vi "value to Rcode.vi"(9 "Manual Range (0)":dbl format="%#_6p", 11 "Function (1: DC Volts)":u16(ring)=1 items=["DC Volts"=1, "AC Volts"=2, "2-Wire Resistance"=3, "4-Wire Resistance"=4, "DC Current"=5, "AC Current"=6, "(AC + DC) Volts"=7, "(AC + DC) Current"=8, "DCV Bch"=12, "Diode"=13, "2-Wire Resistance( Low-Power)"=20, "4-Wire Resistance( Low-Power)"=21, "Continuity"=22, "Frequency"=50]) -> (2 "Range Set Code":string)   [LabVIEW 2020, in "ADCMT7451_ADC.lvlib"]
uses:
  ADCMT7451_ADC.lvlib
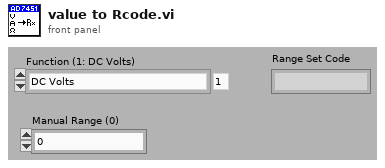
[diagram p1: front panel]
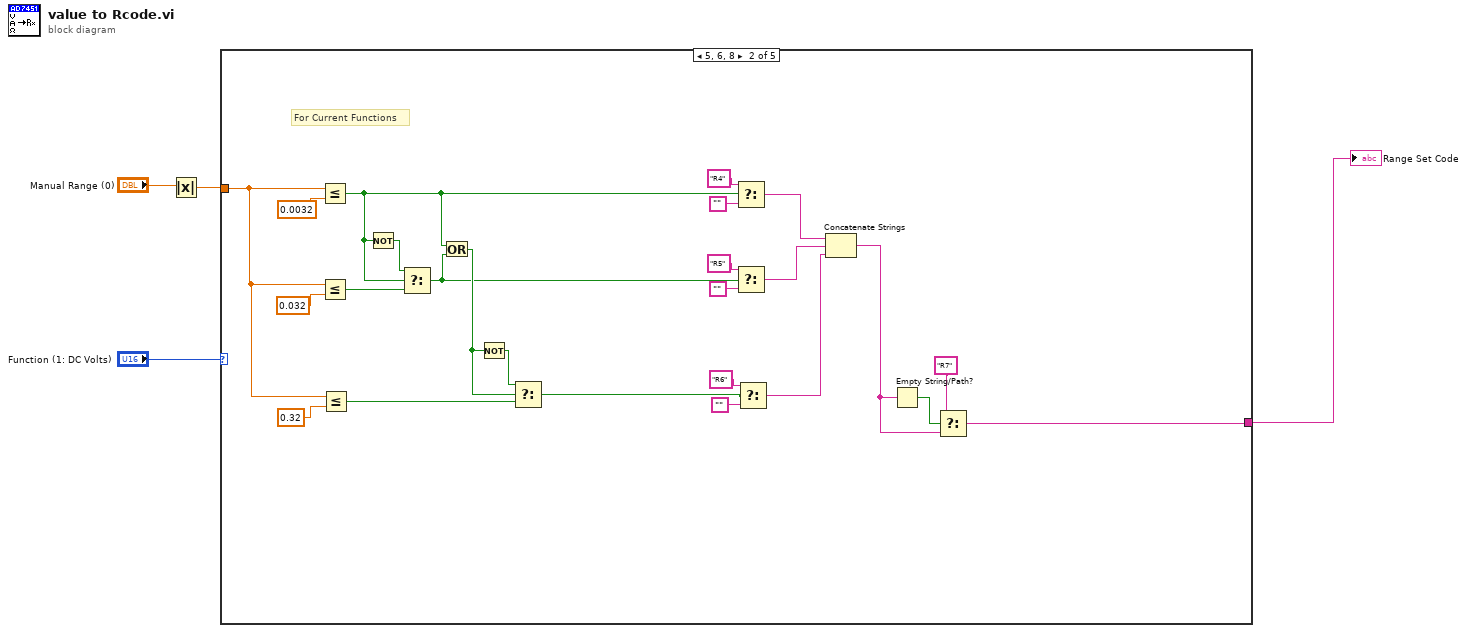
[diagram p0: block diagram]
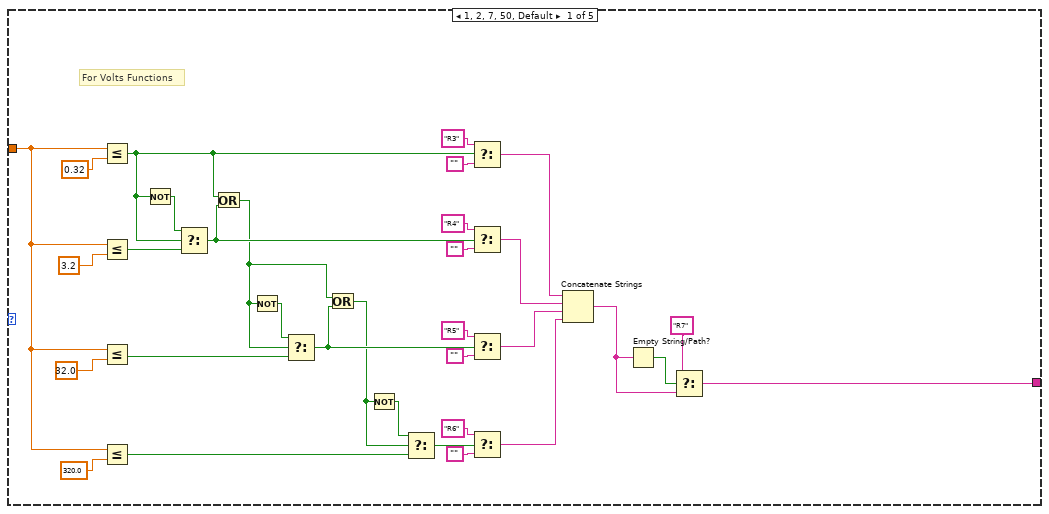
[diagram p2: hidden frame]
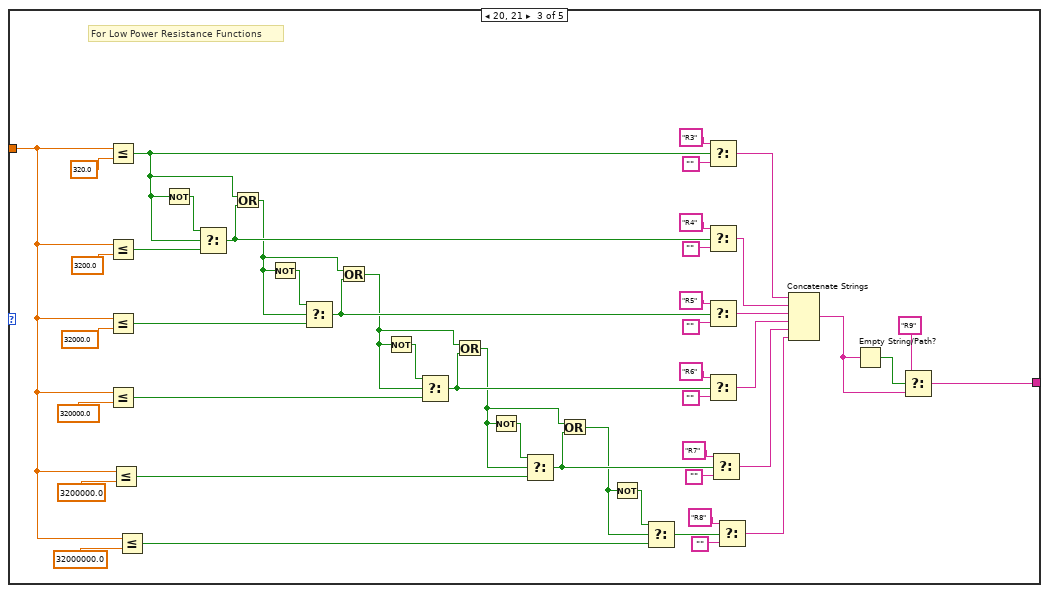
[diagram p3: hidden frame]
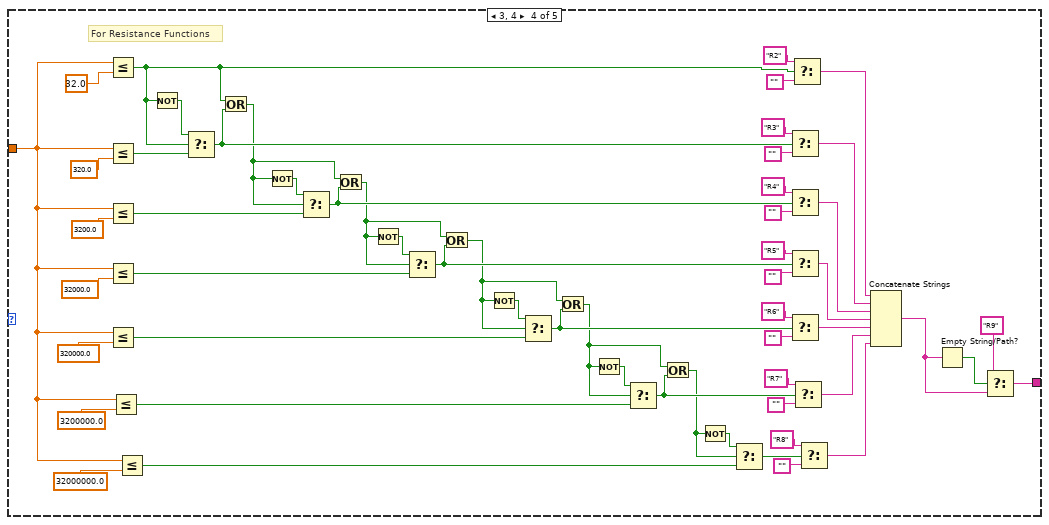
[diagram p4: hidden frame]
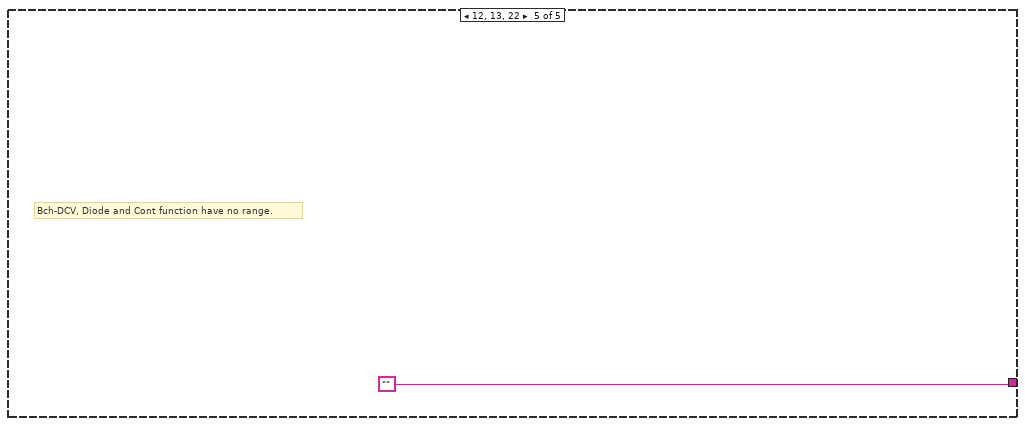
[diagram p5: hidden frame]
diagram:
  n1 = Absolute Value(x="Manual Range (0)") -> (abs(x)=w2:dbl)
  n2 = case shown="5, 6, 8" "Function (1: DC Volts)" {
    tunnel: w2 -> [w25 w42 w64 w121 _]
    tunnel: [w17 w51 w93 w151 ""] -> w3
    frame 1, 2, 7, 50, Default {
      # "For Volts Functions"
      n3 = Less Or Equal?(x=w25, y=0.32) -> (x <= y?=w9:bool)
      n4 = Less Or Equal?(x=w25, y=3.2) -> (x <= y?=w16:bool)
      n5 = Less Or Equal?(x=w25, y=32.0) -> (x <= y?=w13:bool)
      n6 = Less Or Equal?(x=w25, y=320.0) -> (x <= y?=w11:bool)
      n7 = Not(x=w9) -> (.not. x?=w15:bool)
      n8 = Select(t=w15, s=w9, f=w16) -> (s? t:f=w8:bool)
      n9 = Or(x=w9, y=w8) -> (x .or. y?=w5:bool)
      n10 = Not(x=w5) -> (.not. x?=w14:bool)
      n11 = Select(t=w14, s=w5, f=w13) -> (s? t:f=w7:bool)
      n12 = Or(x=w5, y=w7) -> (x .or. y?=w6:bool)
      n13 = Not(x=w6) -> (.not. x?=w12:bool)
      n14 = Select(t=w12, s=w6, f=w11) -> (s? t:f=w10:bool)
      n15 = Select(t="R3", s=w9, f="") -> (s? t:f=w24:string)
      n16 = Select(t="R4", s=w8, f="") -> (s? t:f=w23:string)
      n17 = Select(t="R5", s=w7, f="") -> (s? t:f=w22:string)
      n18 = Select(t="R6", s=w10, f="") -> (s? t:f=w21:string)
      n19 = Concatenate Strings(w24, w23, w22, w21) -> (w18:string)
      n20 = Empty String/Path?(string/path=w18) -> (empty?=w20:bool)
      n21 = Select(t="R7", s=w20, f=w18) -> (s? t:f=w17:string)
    }
    frame 5, 6, 8 {
      # "For Current Functions"
      n22 = Less Or Equal?(x=w42, y=0.0032) -> (x <= y?=w46:bool)
      n23 = Less Or Equal?(x=w42, y=0.032) -> (x <= y?=w49:bool)
      n24 = Less Or Equal?(x=w42, y=0.32) -> (x <= y?=w43:bool)
      n25 = Not(x=w46) -> (.not. x?=w50:bool)
      n26 = Select(t=w50, s=w46, f=w49) -> (s? t:f=w45:bool)
      n27 = Or(x=w46, y=w45) -> (x .or. y?=w47:bool)
      n28 = Not(x=w47) -> (.not. x?=w48:bool)
      n29 = Select(t=w48, s=w47, f=w43) -> (s? t:f=w39:bool)
      n30 = Select(t="R4", s=w46, f="") -> (s? t:f=w56:string)
      n31 = Select(t="R5", s=w45, f="") -> (s? t:f=w55:string)
      n32 = Select(t="R6", s=w39, f="") -> (s? t:f=w38:string)
      n33 = Concatenate Strings(w56, w55, w38) -> (w52:string)
      n34 = Empty String/Path?(string/path=w52) -> (empty?=w54:bool)
      n35 = Select(t="R7", s=w54, f=w52) -> (s? t:f=w51:string)
    }
    frame 20, 21 {
      # "For Low Power Resistance Functions"
      n36 = Less Or Equal?(x=w64, y=320.0) -> (x <= y?=w63:bool)
      n37 = Less Or Equal?(x=w64, y=3200.0) -> (x <= y?=w82:bool)
      n38 = Less Or Equal?(x=w64, y=32000.0) -> (x <= y?=w80:bool)
      n39 = Less Or Equal?(x=w64, y=320000.0) -> (x <= y?=w78:bool)
      n40 = Less Or Equal?(x=w64, y=3200000.0) -> (x <= y?=w74:bool)
      n41 = Less Or Equal?(x=w64, y=32000000.0) -> (x <= y?=w71:bool)
      n42 = Not(x=w63) -> (.not. x?=w83:bool)
      n43 = Select(t=w83, s=w63, f=w82) -> (s? t:f=w77:bool)
      n44 = Or(x=w63, y=w77) -> (x .or. y?=w67:bool)
      n45 = Not(x=w67) -> (.not. x?=w81:bool)
      n46 = Select(t=w81, s=w67, f=w80) -> (s? t:f=w76:bool)
      n47 = Or(x=w67, y=w76) -> (x .or. y?=w66:bool)
      n48 = Not(x=w66) -> (.not. x?=w79:bool)
      n49 = Select(t=w79, s=w66, f=w78) -> (s? t:f=w68:bool)
      n50 = Or(x=w66, y=w68) -> (x .or. y?=w65:bool)
      n51 = Not(x=w65) -> (.not. x?=w75:bool)
      n52 = Select(t=w75, s=w65, f=w74) -> (s? t:f=w73:bool)
      n53 = Or(x=w65, y=w73) -> (x .or. y?=w69:bool)
      n54 = Not(x=w69) -> (.not. x?=w72:bool)
      n55 = Select(t=w72, s=w69, f=w71) -> (s? t:f=w70:bool)
      n56 = Select(t="R3", s=w63, f="") -> (s? t:f=w99:string)
      n57 = Select(t="R4", s=w77, f="") -> (s? t:f=w98:string)
      n58 = Select(t="R5", s=w76, f="") -> (s? t:f=w97:string)
      n59 = Select(t="R6", s=w68, f="") -> (s? t:f=w86:string)
      n60 = Select(t="R7", s=w73, f="") -> (s? t:f=w84:string)
      n61 = Select(t="R8", s=w70, f="") -> (s? t:f=w85:string)
      n62 = Concatenate Strings(w99, w98, w97, w86, w84, w85) -> (w94:string)
      n63 = Empty String/Path?(string/path=w94) -> (empty?=w96:bool)
      n64 = Select(t="R9", s=w96, f=w94) -> (s? t:f=w93:string)
    }
    frame 3, 4 {
      # "For Resistance Functions"
      n65 = Less Or Equal?(x=w121, y=32.0) -> (x <= y?=w115:bool)
      n66 = Less Or Equal?(x=w121, y=320.0) -> (x <= y?=w119:bool)
      n67 = Less Or Equal?(x=w121, y=3200.0) -> (x <= y?=w140:bool)
      n68 = Less Or Equal?(x=w121, y=32000.0) -> (x <= y?=w138:bool)
      n69 = Less Or Equal?(x=w121, y=320000.0) -> (x <= y?=w136:bool)
      n70 = Less Or Equal?(x=w121, y=3200000.0) -> (x <= y?=w132:bool)
      n71 = Less Or Equal?(x=w121, y=32000000.0) -> (x <= y?=w129:bool)
      n72 = Not(x=w115) -> (.not. x?=w120:bool)
      n73 = Select(t=w120, s=w115, f=w119) -> (s? t:f=w116:bool)
      n74 = Or(x=w115, y=w116) -> (x .or. y?=w114:bool)
      n75 = Not(x=w114) -> (.not. x?=w141:bool)
      n76 = Select(t=w141, s=w114, f=w140) -> (s? t:f=w135:bool)
      n77 = Or(x=w114, y=w135) -> (x .or. y?=w125:bool)
      n78 = Not(x=w125) -> (.not. x?=w139:bool)
      n79 = Select(t=w139, s=w125, f=w138) -> (s? t:f=w134:bool)
      n80 = Or(x=w125, y=w134) -> (x .or. y?=w124:bool)
      n81 = Not(x=w124) -> (.not. x?=w137:bool)
      n82 = Select(t=w137, s=w124, f=w136) -> (s? t:f=w126:bool)
      n83 = Or(x=w124, y=w126) -> (x .or. y?=w123:bool)
      n84 = Not(x=w123) -> (.not. x?=w133:bool)
      n85 = Select(t=w133, s=w123, f=w132) -> (s? t:f=w131:bool)
      n86 = Or(x=w123, y=w131) -> (x .or. y?=w127:bool)
      n87 = Not(x=w127) -> (.not. x?=w130:bool)
      n88 = Select(t=w130, s=w127, f=w129) -> (s? t:f=w128:bool)
      n89 = Select(t="R3", s=w116, f="") -> (s? t:f=w113:string)
      n90 = Select(t="R4", s=w135, f="") -> (s? t:f=w156:string)
      n91 = Select(t="R5", s=w134, f="") -> (s? t:f=w155:string)
      n92 = Select(t="R6", s=w126, f="") -> (s? t:f=w144:string)
      n93 = Select(t="R2", s=w115, f="") -> (s? t:f=w112:string)
      n94 = Select(t="R7", s=w131, f="") -> (s? t:f=w142:string)
      n95 = Select(t="R8", s=w128, f="") -> (s? t:f=w143:string)
      n96 = Concatenate Strings(w112, w113, w156, w155, w144, w142, w143) -> (w152:string)
      n97 = Empty String/Path?(string/path=w152) -> (empty?=w154:bool)
      n98 = Select(t="R9", s=w154, f=w152) -> (s? t:f=w151:string)
    }
    frame 12, 13, 22 {
      # "Bch-DCV, Diode and Cont function have no range."
    }
  }
  "Range Set Code" <- w3
